vi "Power Spectrum to Waveform.vi"(1 "Power Spectrum":cluster{"f0":dbl, "df":dbl, "magnitude":dbl[]}) -> (0 "Waveform":waveform(dbl))   [LabVIEW 2011]
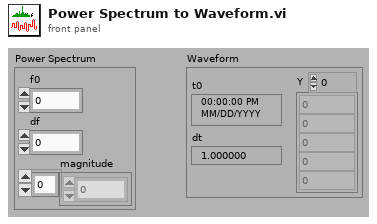
[diagram p1: front panel]
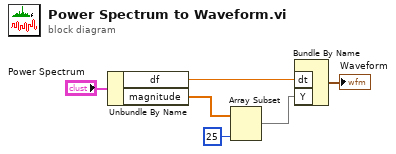
[diagram p0: block diagram]
diagram:
  n1 = Unbundle By Name("Power Spectrum") -> ("df"=w4:dbl, "magnitude"=w3:dbl[])
  n2 = Array Subset(array=w3, length=25) -> (w1:dbl[])  [unwired: 1 in]
  n3 = Bundle By Name("dt"=w4, "Y"=w1) -> (→"Waveform":waveform(dbl))  [unwired: 1 in]
